vi "LV to JSON Test.vi"() -> ()   [LabVIEW 2015]
uses:
  lib/JSON.lvlib
panel:
  out "TOML String":string
  in  "Data":T1={"Number"=0.0, "Array"=[[{"Boolean"=FALSE}, {"Boolean"=FALSE}], [{"Boolean"=TRUE}, {"Boolean"=FALSE}]], "Object"={"String"=""}}
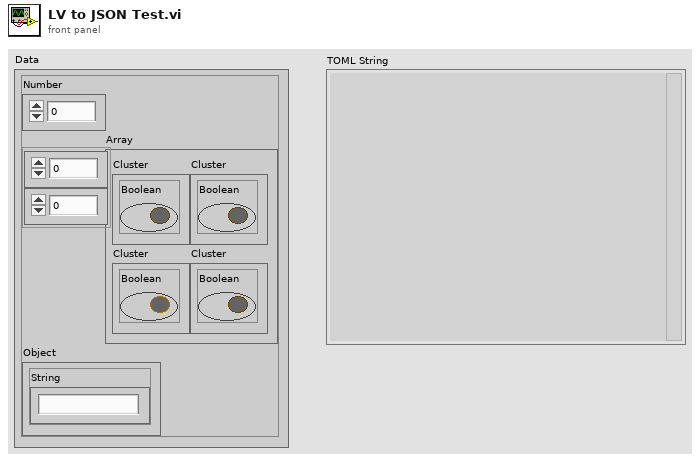
[diagram p1: front panel]
types:
  T1 = cluster{"Number":dbl, "Array":cluster{"Boolean":bool}[][], "Object":cluster{"String":string}}
  T2 = typedef "JSON.lvlib/JSON Value.ctl" = cluster{"\\type":enum16{"Object", "Array", "String", "Number", "Boolean", "Null"}, "ÿýÿýÿýÿýÿýÿþÿýÿýÿý&LV-JSON.lvlib:JSON Name-Value Pair.ctlÿýÿýÿýÿýÿýÿþÿýÿýÿýLV-JSON.lvlib:JSON Value.ctl":variant}
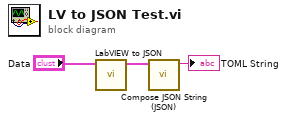
[diagram p0: block diagram]
diagram:
  n1 = call "LabVIEW to JSON.vi"("LV Value"="Data") -> ("JSON Value"=w2:T2)  [unwired: 9 in, 1 out]
  n2 = call "Compose JSON String (JSON).vi"("Value"=w2) -> ("String"=→"TOML String":string)  [unwired: 9 in, 1 out]
